vi "compare middle sectors.vi"(1 "Right":u16[](array[numeric]), 2 "Left":u16[](array[numeric])) -> (0 "Middle subsectors values":u16[](array[numeric]))   [LabVIEW 2009]
doc: "This subvi merges the two overlapping sectors\nby taking the lower sick value for each sector."
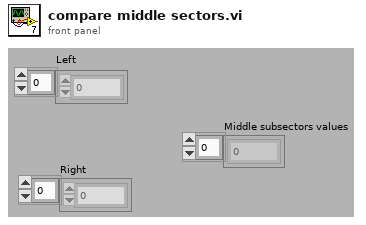
[diagram p1: front panel]
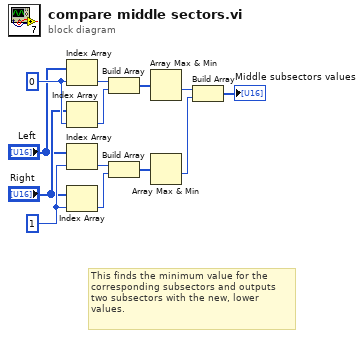
[diagram p0: block diagram]
diagram:
  w12 = 1 ("index")
  w13 = 0 ("index")
  # "This finds the minimum value for the \ncorresponding subsectors and outputs\ntwo subsectors with the new, lower\nvalues."
  n1 = Index Array(array="Left", index=w13) -> (element=w9:u16)
  n2 = Index Array(array="Right", index=w13) -> (element=w8:u16)
  n3 = Index Array(array="Left", index=w12) -> (element=w3:u16)
  n4 = Index Array(array="Right", index=w12) -> (element=w4:u16)
  n5 = Build Array(w9, w8) -> (w7:u16[])
  n6 = Build Array(w3, w4) -> (w5:u16[])
  n7 = Array Max & Min(array=w7) -> (min value=w6:u16)  [unwired: 3 out]
  n8 = Array Max & Min(array=w5) -> (min value=w2:u16)  [unwired: 3 out]
  n9 = Build Array(w6, w2) -> (→"Middle subsectors values":u16[])
